vi "LRPTOM.vi"() -> ()   [LabVIEW 2013]
uses:
  Classes/OSSP_Problem.lvclass
  Classes/GanntChart_Class/Operation to Machine Job Tuple.vi
  <vilib>/regexp/Match Regular Expression.xnode
  Classes/GanntChart.lvclass
panel:
  out "Due Dates":u16[](array[numeric])
  out "max value":u16
  out "Operation List":i32[](array[numeric])
  out "Priority List":string[](array[string])
  out "Array":u16[](array[numeric])
  out "Remaining Processing Times 2":u16[][](array[numeric])
  out "output array":u16[][](array[numeric])
  out "Processing Times":u16[][](array[numeric])
  out "Remaining Processing Times":u16[][](array[numeric])
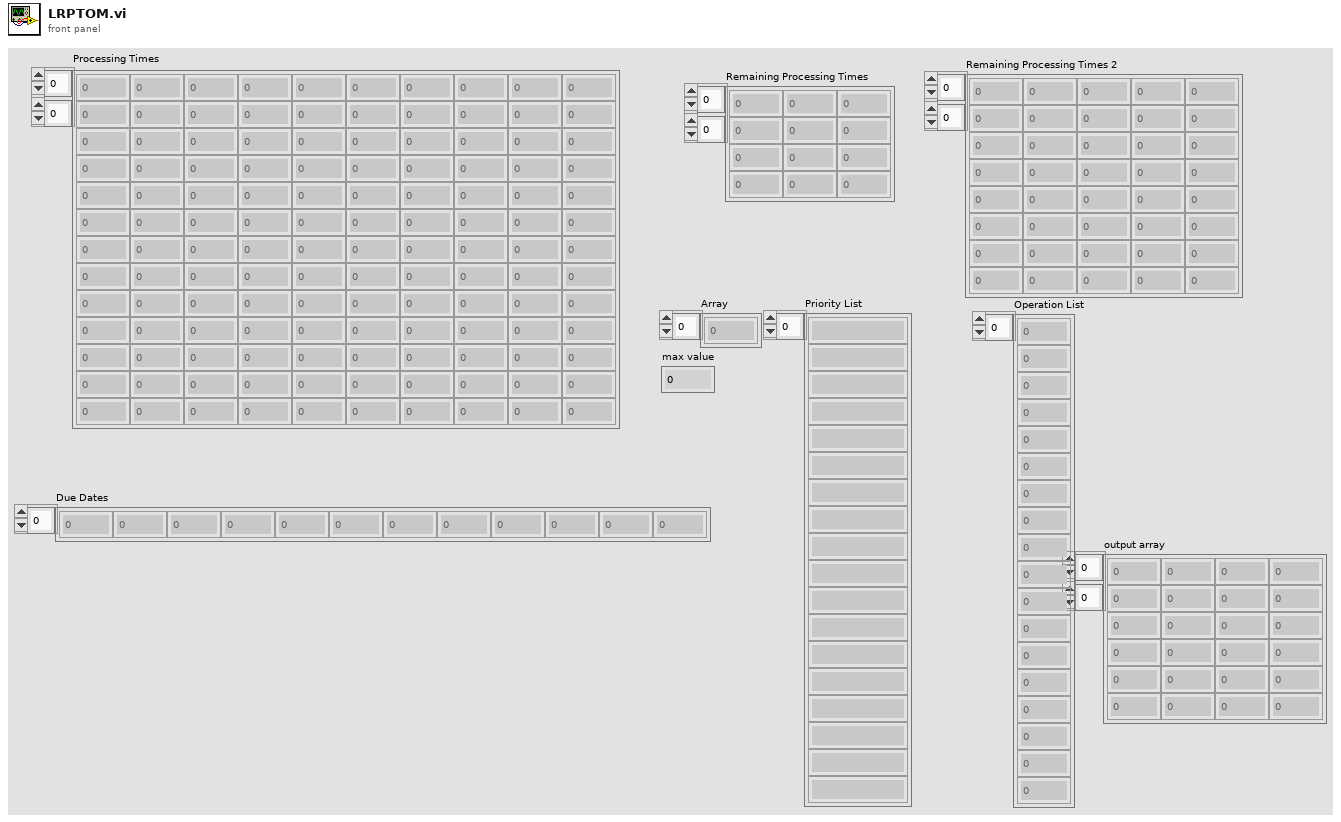
[diagram p1: front panel]
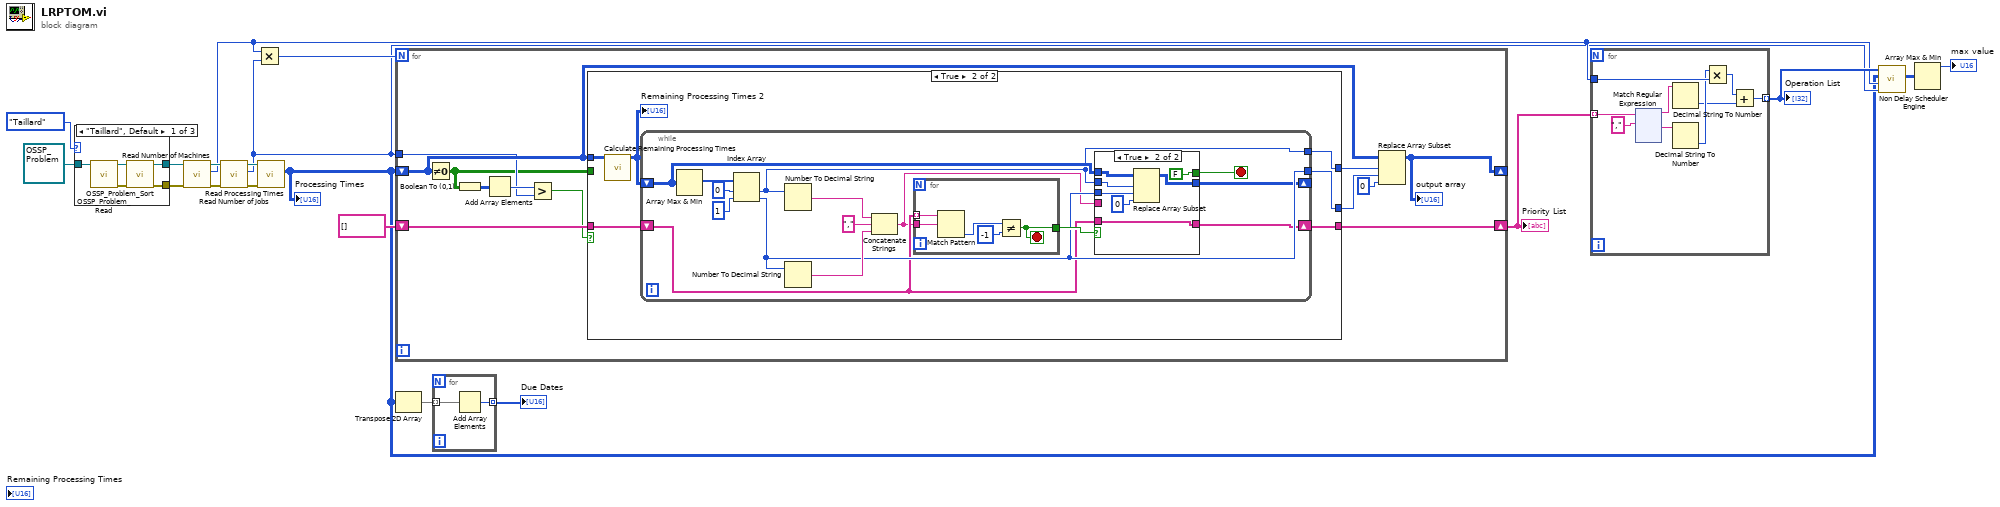
[diagram p0: block diagram]
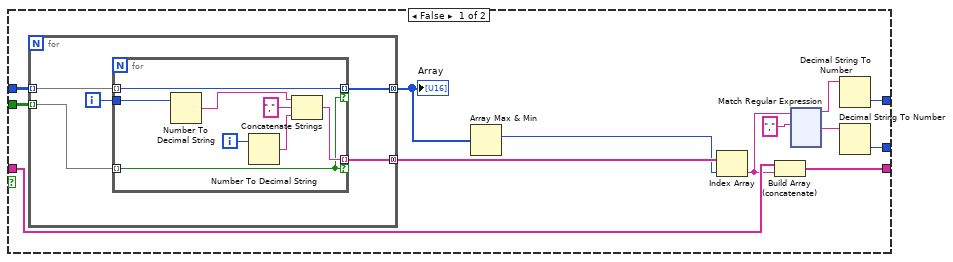
[diagram p2: hidden frame]
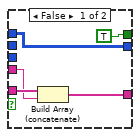
[diagram p3: hidden frame]
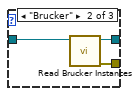
[diagram p4: hidden frame]
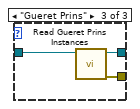
[diagram p5: hidden frame]
diagram:
  n1 = case shown="\"Taillard\", Default" enum16{"Taillard", "Brucker", "Gueret Prins"}."Taillard" {
    tunnel: [w22 w27 w30] -> w4
    tunnel: refnum<class "OSSP_Problem.lvclass"> refnum ("OSSP_Problem out") -> [w24 w26 w29]
    tunnel: [w20 w25 w28] -> w3
    frame "Taillard", Default {
      n2 = call "OSSP_Problem_Read.vi"("OSSP_Problem.lvclass In"=w24) -> ("error out"=w21:errorcluster, "OSSP_Problem.lvclass Out"=w23:refnum<class "OSSP_Problem.lvclass">)  [unwired: 9 in]
      n3 = call "OSSP_Problem_Sort.vi"("error in (no error)"=w21, "OSSP_Problem.lvclass In"=w23) -> ("error out"=w20:errorcluster, "OSSP_Problem.lvclass Out"=w22:refnum<class "OSSP_Problem.lvclass">)  [unwired: 8 in]
    }
    frame "Brucker" {
      n4 = call "Read Brucker Instances.vi"("OSSP_Problem in"=w26) -> ("error out"=w25:errorcluster, "OSSP_Problem out"=w27:refnum<class "OSSP_Problem.lvclass">)  [unwired: 9 in]
    }
    frame "Gueret Prins" {
      n5 = call "Read Gueret Prins Instances.vi"("OSSP_Problem in"=w29) -> ("error out"=w28:errorcluster, "OSSP_Problem out"=w30:refnum<class "OSSP_Problem.lvclass">)  [unwired: 9 in]
    }
  }
  n6 = call-dynamic "Read Number of Machines.vi"("error in (no error)"=w3, "OSSP_Problem in"=w4) -> ("error out"=w17:errorcluster, "Number of Machines"=w9:i32, "OSSP_Problem out"=w19:refnum<class "OSSP_Problem.lvclass">)  [unwired: 7 in]
  n7 = call-dynamic "Read Number of Jobs.vi"("error in (no error)"=w17, "OSSP_Problem in"=w19) -> ("error out"=w16:errorcluster, "Number of Jobs"=w8:i32, "OSSP_Problem out"=w18:refnum<class "OSSP_Problem.lvclass">)  [unwired: 7 in]
  n8 = Multiply(x=w9, y=w8) -> (x*y=w13:i32)
  n9 = call-dynamic "Read Processing Times.vi"("error in (no error)"=w16, "OSSP_Problem in"=w18) -> ("Processing Times"=w2:u16[][])  [unwired: 7 in, 2 out]
  "Processing Times" <- w2
  n10 = for {
    N: w13 -> [_]
    shift-right: [w41] -> _
    shift-left: w2 -> [w36]
    shift-right: [w37] -> w11
    shift-left: string[] [] -> [w38]
    tunnel: w8 -> [w33]
    n11 = Not Equal To 0?(x=w36) -> (x != 0?=w31:bool[][])
    n12 = Boolean To (0,1)(Boolean=w31) -> (0, 1=w35:i16[][])
    n13 = Add Array Elements(numeric array=w35) -> (sum=w34:i16)
    n14 = Greater?(x=w34, y=w33) -> (0:w32:bool)
    n15 = case shown="True" w32 {
      tunnel: w36 -> [w55 w187]
      tunnel: [w43 w186] -> w40
      tunnel: [w44 w185] -> w39
      tunnel: w38 -> [w47 w184]
      tunnel: [w45 w183] -> w37
      tunnel: w31 -> [w54 _]
      frame False {
        n16 = for {
          tunnel: w55 -> [w174] mode=indexing
          tunnel: w54 -> [w173] mode=indexing
          tunnel: [w172] -> w53 mode=concatenating
          tunnel: [w170] -> w52 mode=concatenating
          i -> [w171]
          n17 = for {
            tunnel: w174 -> [w182] mode=indexing
            tunnel: w173 -> [w175] mode=indexing
            tunnel: [w182] -> w172 mode=indexing if=w175
            tunnel: w171 -> [w181]
            tunnel: [w176] -> w170 mode=indexing if=w175
            i -> [w180]
            n18 = Number To Decimal String(number=w181) -> (decimal integer string=w179:string)  [unwired: 1 in]
            n19 = Number To Decimal String(number=w180) -> (decimal integer string=w177:string)  [unwired: 1 in]
            n20 = Concatenate Strings(w179, "," ("string"), w177) -> (w176:string)
          }
        }
        "Array" <- w53
        n21 = Array Max & Min(array=w53) -> (max index (indices)=w51:i32)  [unwired: 3 out]
        n22 = Index Array(array=w52, index=w51) -> (element=w46:string)
        n23 = Build Array (concatenate)(w47, w46) -> (w45:string[])
        n24 = xnode "Match Regular Expression"("input string"=w46, "regular expression"=",") -> ("before match"=w49:string, "after match"=w48:string)  [unwired: 4 in, 3 out]
        n25 = Decimal String To Number(string=w49) -> (number=w43:i32)  [unwired: 2 in, 1 out]
        n26 = Decimal String To Number(string=w48) -> (number=w44:i32)  [unwired: 2 in, 1 out]
      }
      frame True {
        n27 = call "Calculate Remaining Processing Times.vi"("Processing Times"=w187) -> ("Remaining Processing Times"=w188:u16[][])  [unwired: 10 in]
        "Remaining Processing Times 2" <- w188
        n28 = while {
          tunnel: [w195] -> w186
          tunnel: [w194] -> w185
          shift-right: [w193] -> _
          shift-left: w188 -> [w196]
          shift-right: [w190] -> w183
          shift-left: w184 -> [w192]
          stop <- w189 stop-if-true
          n29 = Array Max & Min(array=w196) -> (max index (indices)=w203:i32[])  [unwired: 3 out]
          n30 = Index Array(array=w203, index #1=0 ("index"), index #2=1 ("index")) -> (element #1=w195:i32, element #2=w194:i32)
          n31 = Number To Decimal String(number=w195) -> (decimal integer string=w200:string)  [unwired: 1 in]
          n32 = Number To Decimal String(number=w194) -> (decimal integer string=w199:string)  [unwired: 1 in]
          n33 = Concatenate Strings(w200, "," ("string"), w199) -> (w191:string)
          n34 = for {
            tunnel: w192 -> [w220] mode=indexing
            tunnel: w191 -> [w219]
            tunnel: [w216] -> w197
            stop <- w216 stop-if-true
            n35 = Match Pattern(string=w220, regular expression=w219) -> (offset past match=w218:i32)  [unwired: 1 in, 3 out]
            n36 = Not Equal?(x=w218, y=-1) -> (x != y?=w216:bool)
          }
          n37 = case shown="True" w197 {
            tunnel: w196 -> [w205 w215]
            tunnel: w195 -> [_ w214]
            tunnel: w194 -> [_ w213]
            tunnel: [w205 w211] -> w193
            tunnel: w192 -> [w208 w210]
            tunnel: w191 -> [w207 _]
            tunnel: [w206 w210] -> w190
            tunnel: [TRUE FALSE] -> w189
            frame False {
              n38 = Build Array (concatenate)(w208, w207) -> (w206:string[])
            }
            frame True {
              n39 = Replace Array Subset(array=w215, new element=u16 0 ("new element/subarray"), index (row)=w214, index (col)=w213) -> (w211:u16[][])
            }
          }
        }
      }
    }
    n40 = Replace Array Subset(array=w36, new element=u16 0 ("new element/subarray"), index (row)=w40, index (col)=w39) -> (w41:u16[][])
    "output array" <- w41
  }
  "Priority List" <- w11
  n41 = Transpose 2D Array(2D array=w2) -> (transposed array=w5:u16[][])
  n42 = for {
    tunnel: w5 -> [w222] mode=indexing
    tunnel: [w221] -> w1 mode=indexing
    n43 = Add Array Elements(numeric array=w222) -> (sum=w221:u16)
  }
  "Due Dates" <- w1
  n44 = for {
    tunnel: w11 -> [w231] mode=indexing
    tunnel: w9 -> [w227]
    tunnel: [w223] -> w10 mode=indexing
    n45 = xnode "Match Regular Expression"("input string"=w231, "regular expression"=",") -> ("before match"=w229:string, "after match"=w228:string)  [unwired: 4 in, 3 out]
    n46 = Decimal String To Number(string=w229) -> (number=w224:i32)  [unwired: 2 in, 1 out]
    n47 = Decimal String To Number(string=w228) -> (number=w226:i32)  [unwired: 2 in, 1 out]
    n48 = Multiply(x=w226, y=w227) -> (x*y=w225:i32)
    n49 = Add(x=w225, y=w224) -> (x+y=w223:i32)
  }
  "Operation List" <- w10
  n50 = call "Non Delay Scheduler Engine.vi"("Number of  Jobs"=w8, "Number of Machines"=w9, "Processing Times"=w2, "Schedule"=w10) -> ("Completion Times"=w7:u16[][])  [unwired: 3 in, 4 out]
  n51 = Array Max & Min(array=w7) -> (max value=→"max value":u16)  [unwired: 3 out]
